vi "Modbus Status Bitmap System Faults.vi"(4 "Gen Start Fault":bool=TRUE, 6 "Manual Shutdown":bool=TRUE, 7 "Gen Data Array":T1[](array[typedef]) {"TotalFuel(L)" format="%.2f"; "FuelRate(L/H)" format="%.2f"; "ApparentPower(VA)" format="%.2f"; "BattVoltage(V)" format="%.2f"; "Freq(Hz)" format="%.2f"; "RunHours(hr)" format="%.2f"; "PowerFactor" format="%.2f"; "ReactivePower(VAR)" format="%.2f"; "ActivePower(W)" format="%.2f"}, 8 "Error In":errorcluster, 9 "FPGA Data In":T2 {"SSG Active Current" format="%2.1f"; "PV Reactive Power (L1)" format="%2.1f"; "PV Reactive Power (L2)" format="%2.1f"; "PV Total Reactive Power" format="%2.1f"; "Gen Reactive Power (L1)" format="%2.1f"; "Gen Reactive Power (L2)" format="%2.1f"; "Gen Total Reactive Power" format="%2.1f"; "SSG Reactive Power (L1)" format="%2.1f"; "SSG Reactive Power (L2)" format="%2.1f"; "SSG Total Reactive Power" format="%2.1f"; "PV Total Current" format="%2.1f"; "PV Total Voltage" format="%2.1f"; "PV Active Power (L1)" format="%2.1f"; "PV Active Power (L2)" format="%2.1f"; "PV App Power (L1)" format="%2.1f"; "PV App Power (L2)" format="%2.1f"; "PV Total Active Power" format="%2.1f"; "PV Total App Power" format="%2.1f"; "PV Arms (L1)" format="%2.1f"; "PV Arms (L2)" format="%2.1f"; "PV Vrms (L1)" format="%2.1f"; "PV Vrms (L2)" format="%2.1f"; "Gen Total Current" format="%2.1f"; "SSG Total Current" format="%2.1f"; "Gen Total Voltage" format="%2.1f"; "SSG Total Voltage" format="%2.1f"; "Gen Active Power (L1)" format="%2.1f"; "Gen Active Power (L2)" format="%2.1f"; "SSG Active Power (L1)" format="%2.1f"; "SSG Active Power (L2)" format="%2.1f"; "Gen App Power (L1)" format="%2.1f"; "Gen App Power (L2)" format="%2.1f"; "SSG App Power (L1)" format="%2.1f"; "SSG App Power (L2)" format="%2.1f"; "Gen Total Active Power" format="%2.1f"; "Gen Total App Power" format="%2.1f"; "Gen Arms (L1)" format="%2.1f"; "Gen Arms (L2)" format="%2.1f"; "Gen Vrms (L1)" format="%2.1f"; "Gen Vrms (L2)" format="%2.1f"; "SSG Total Active Power" format="%2.1f"; "SSG Total App Power" format="%2.1f"; "SSG Arms (L1)" format="%2.1f"; "SSG Arms (L2)" format="%2.1f"; "SSG Vrms (L1)" format="%2.1f"; "SSG Vrms (L2)" format="%2.1f"}, 10 "PC Data In":T3 {"Alarms 2" format="%016b"; "Faults 2" format="%016b"; "Alarms 1" format="%016b"; "Faults 1" format="%016b"; "Contactor FB" format="%.0b"; "DC Voltage SP" format="%2.1f"; "Clear Faults SP" format="%.0b"; "Neutral Current" format="%2.1f"; "AC Current - L2" format="%2.1f"; "AC Voltage - L2" format="%2.1f"; "Temperature" format="%2.1f"; "DC Voltage" format="%2.1f"; "AC Current SP" format="%2.1f"; "AC Voltage SP" format="%2.1f"; "Frequency SP" format="%2.1f"; "AC Frequency" format="%2.1f"; "AC Current - L1" format="%2.1f"; "AC Voltage- L1" format="%2.1f"}, 11 "ES System Data In":T5={"Voltage"=0.0, "Current"=0.0, "SOC Avg"=0.0, "Faults"=0, "Alarms"=0, "# Strings"=0, "Max Temp"=0, "Min Temp"=0, "Max Cell Voltage"=0.0, "Min Cell Voltage"=0.0, "Energy Capacity"=0.0, "Energy Remaining"=0.0, "SOC Min"=0.0, "SOC Max"=0.0, "ES Fault"=FALSE, "String Select"=enum."3 Strings", "ES Com Fault"=FALSE, "SOH Avg"=0.0}) -> (0 "Error Out":errorcluster, 1 "PV Faults":i16, 2 "Controller Faults":i16, 3 "System Faults":i16)   [LabVIEW 2014]
uses:
  Controls/ES System Data.ctl
  Controls/StringSelector.ctl
  Controls/PC Data.ctl
  Controls/MicroZed Config Op Mode.ctl
  Controls/FPGA Data.ctl
  Controls/Gen Data.ctl
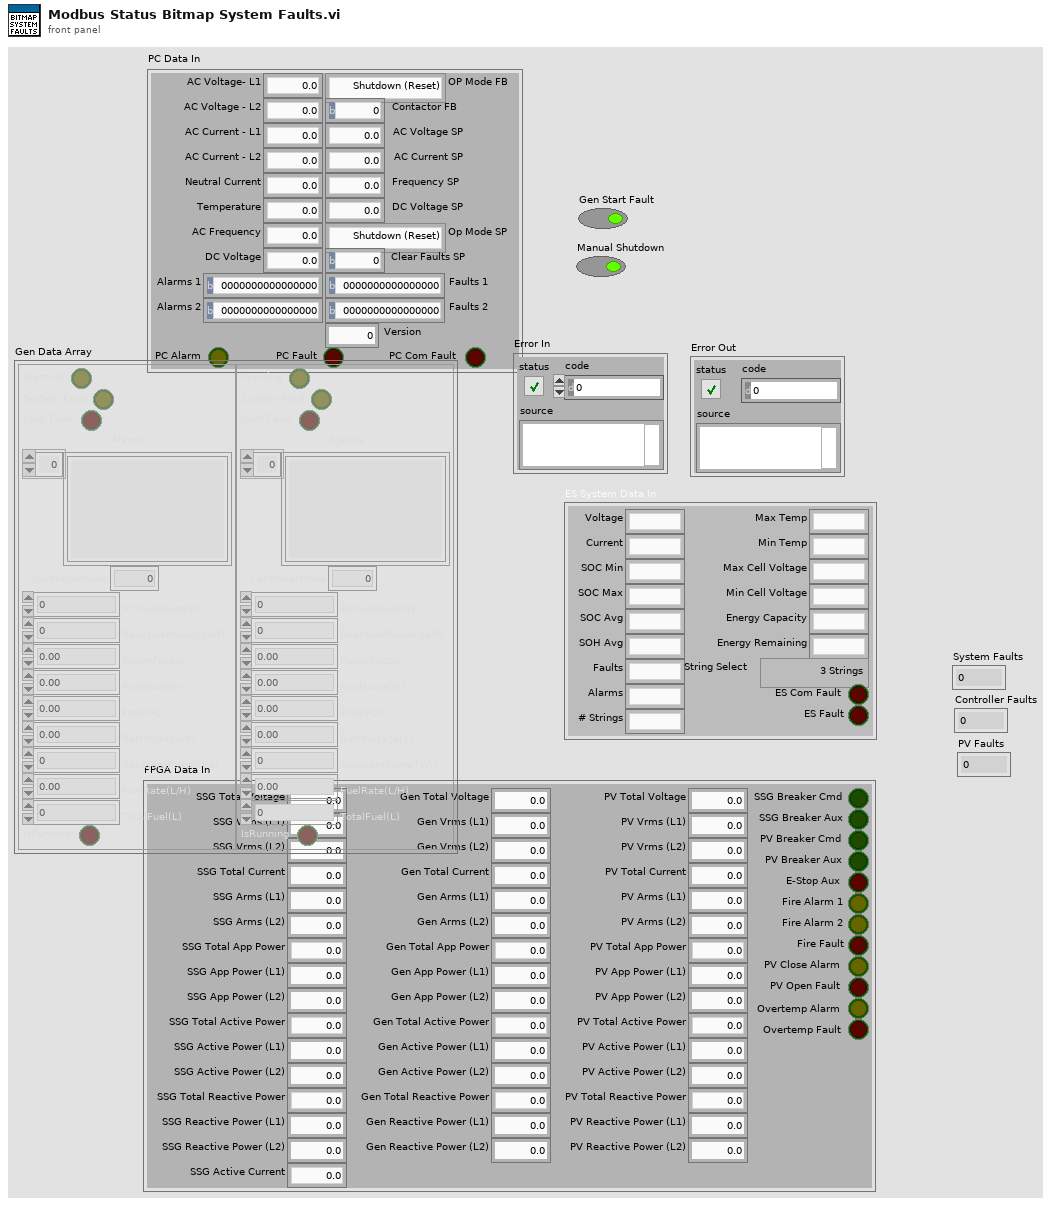
[diagram p1: front panel]
types:
  T1 = typedef "Gen Data.ctl" = cluster{"Warning":bool, "System Fault":bool, "Com Fault":bool, "Alarms":string[], "ControllerMode":u16, "ActivePower(W)":i32, "ReactivePower(VAR)":i32, "PowerFactor":dbl, "RunHours(hr)":dbl, "Freq(Hz)":dbl, "BattVoltage(V)":dbl, "ApparentPower(VA)":i32, "FuelRate(L/H)":dbl, "TotalFuel(L)":u32, "IsRunning":bool}
  T2 = typedef "FPGA Data.ctl" = cluster{"Gen Total Voltage":dbl, "Gen Vrms (L1)":dbl, "Gen Vrms (L2)":dbl, "Gen Total Current":dbl, "Gen Arms (L1)":dbl, "Gen Arms (L2)":dbl, "Gen Total App Power":dbl, "Gen App Power (L1)":dbl, "Gen App Power (L2)":dbl, "Gen Total Active Power":dbl, "Gen Active Power (L1)":dbl, "Gen Active Power (L2)":dbl, "Gen Total Reactive Power":dbl, "Gen Reactive Power (L1)":dbl, "Gen Reactive Power (L2)":dbl, "SSG Total Voltage":dbl, "SSG Vrms (L1)":dbl, "SSG Vrms (L2)":dbl, "SSG Total Current":dbl, "SSG Arms (L1)":dbl, "SSG Arms (L2)":dbl, "SSG Total App Power":dbl, "SSG App Power (L1)":dbl, "SSG App Power (L2)":dbl, "SSG Total Active Power":dbl, "SSG Active Power (L1)":dbl, "SSG Active Power (L2)":dbl, "SSG Total Reactive Power":dbl, "SSG Reactive Power (L1)":dbl, "SSG Reactive Power (L2)":dbl, "PV Total Voltage":dbl, "PV Vrms (L1)":dbl, "PV Vrms (L2)":dbl, "PV Total Current":dbl, "PV Arms (L1)":dbl, "PV Arms (L2)":dbl, "PV Total App Power":dbl, "PV App Power (L1)":dbl, "PV App Power (L2)":dbl, "PV Total Active Power":dbl, "PV Active Power (L1)":dbl, "PV Active Power (L2)":dbl, "PV Total Reactive Power":dbl, "PV Reactive Power (L1)":dbl, "PV Reactive Power (L2)":dbl, "SSG Breaker Cmd":bool, "SSG Breaker Aux":bool, "PV Breaker Cmd":bool, "PV Breaker Aux":bool, "E-Stop Aux":bool, "Fire Alarm 1":bool, "Fire Alarm 2":bool, "Fire Fault":bool, "PV Close Alarm":bool, "SSG Active Current":dbl, "Overtemp Alarm":bool, "Overtemp Fault":bool, "PV Open Fault":bool}
  T3 = typedef "PC Data.ctl" = cluster{"AC Voltage- L1":dbl, "AC Voltage - L2":dbl, "AC Current - L1":dbl, "AC Current - L2":dbl, "Neutral Current":dbl, "Temperature":dbl, "AC Frequency":dbl, "DC Voltage":dbl, "AC Voltage SP":dbl, "AC Current SP":dbl, "Frequency SP":dbl, "Op Mode SP":T4, "Clear Faults SP":u16, "PC Com Fault":bool, "PC Fault":bool, "DC Voltage SP":dbl, "OP Mode FB":T4, "Contactor FB":u16, "Faults 1":u16, "Alarms 1":u16, "Faults 2":u16, "Alarms 2":u16, "PC Alarm":bool, "Version":u16}
  T4 = typedef "MicroZed Config Op Mode.ctl" = enum16{"Shutdown (Reset)", "Startup", "Idle", "Voltage Mode", "Current Mode", "Fault", "OL Voltage (Debug)", "No Data"}
  T5 = typedef "ES System Data.ctl" = cluster{"Voltage":sgl, "Current":sgl, "SOC Avg":sgl, "Faults":u16, "Alarms":u16, "# Strings":u16, "Max Temp":i16, "Min Temp":i16, "Max Cell Voltage":sgl, "Min Cell Voltage":sgl, "Energy Capacity":sgl, "Energy Remaining":sgl, "SOC Min":sgl, "SOC Max":sgl, "ES Fault":bool, "String Select":T6, "ES Com Fault":bool, "SOH Avg":sgl}
  T6 = typedef "StringSelector.ctl" = enum16{"1 String (1)", "1 String (2)", "1 String (3)", "2 Strings (1 2)", "2 Strings (2 3)", "2 Strings (1 3)", "3 Strings"}
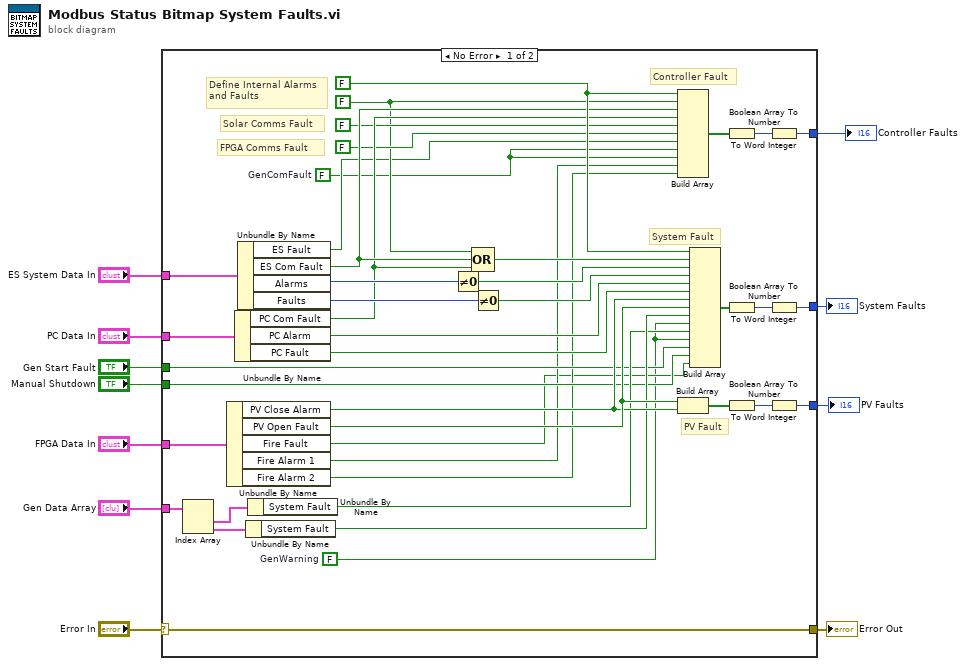
[diagram p0: block diagram]
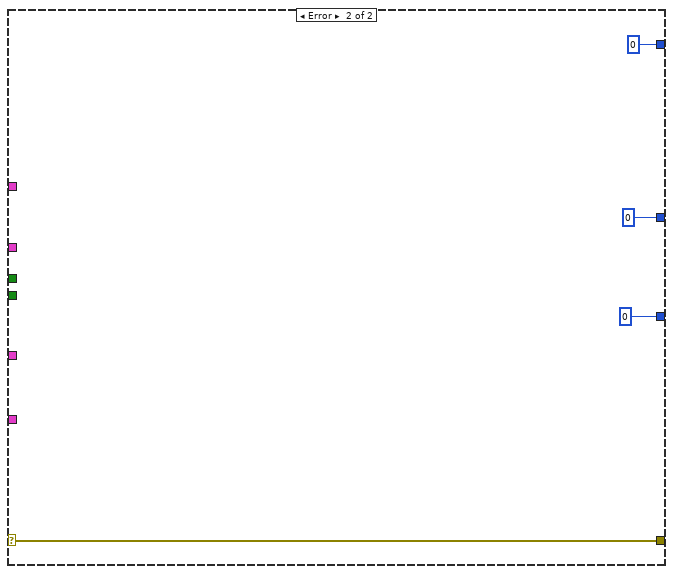
[diagram p2: hidden frame]
diagram:
  n1 = case shown="No Error" "Error In" {
    selector: "Error In" -> [w52 w55]
    tunnel: [w52 w55] -> w10
    tunnel: "FPGA Data In" -> [w45 _]
    tunnel: "PC Data In" -> [w46 _]
    tunnel: "ES System Data In" -> [w51 _]
    tunnel: "Gen Data Array" -> [w44 _]
    tunnel: [w30 i16 0] -> w4
    tunnel: [w29 i16 0] -> w5
    tunnel: [w24 i16 0] -> w3
    tunnel: "Manual Shutdown" -> [w18 _]
    tunnel: "Gen Start Fault" -> [w17 _]
    frame No Error {
      w13 = FALSE  # GenComFault
      w12 = FALSE  # GenWarning
      w35 = FALSE ("element")
      w41 = FALSE ("element")
      # "PV Fault"
      # "System Fault"
      # "Controller Fault"
      # "FPGA Comms Fault"
      # "Solar Comms Fault"
      # "Define Internal Alarms\nand Faults"
      n2 = Index Array(array=w44) -> (element #1=w43:T1, element #2=w42:T1)  [unwired: 2 in]
      n3 = Unbundle By Name(w45) -> ("PV Close Alarm"=w27:bool, "PV Open Fault"=w28:bool, "Fire Fault"=w14:bool, "Fire Alarm 1"=w16:bool, "Fire Alarm 2"=w15:bool)
      n4 = Unbundle By Name(w46) -> ("PC Com Fault"=w38:bool, "PC Alarm"=w21:bool, "PC Fault"=w22:bool)
      n5 = Unbundle By Name(w51) -> ("ES Fault"=w23:bool, "ES Com Fault"=w39:bool, "Alarms"=w50:u16, "Faults"=w49:u16)
      n6 = Unbundle By Name(w42) -> ("System Fault"=w20:bool)
      n7 = Unbundle By Name(w43) -> ("System Fault"=w19:bool)
      n8 = Not Equal To 0?(x=w50) -> (x != 0?=w48:bool)
      n9 = Compound Arithmetic op=OR(w35, w39, w38) -> (w40:bool)
      n10 = Not Equal To 0?(x=w49) -> (x != 0?=w47:bool)
      n11 = Build Array(w41, w35, w39, w38, FALSE ("element"), FALSE ("element"), w23, w13, w13, w16, w15) -> (w34:bool[])
      n12 = Build Array(w28, w27) -> (w25:bool[])
      n13 = Build Array(w41, w40, w48, w47, w21, w22, w27, w28, w20, w12, w19, w12, w17, w18, w14) -> (w33:bool[])
      n14 = Boolean Array To Number(Boolean array=w34) -> (number=w32:u32)
      n15 = Boolean Array To Number(Boolean array=w33) -> (number=w31:u32)
      n16 = Boolean Array To Number(Boolean array=w25) -> (number=w26:u32)
      n17 = To Word Integer(number=w32) -> (16bit integer=w30:i16)
      n18 = To Word Integer(number=w31) -> (16bit integer=w29:i16)
      n19 = To Word Integer(number=w26) -> (16bit integer=w24:i16)
    }
    frame Error {
    }
  }
  "Error Out" <- w10
  "System Faults" <- w5
  "Controller Faults" <- w4
  "PV Faults" <- w3
